vi "vi tree.vi"   [LabVIEW 2020, in "stream_custom_cluster.lvclass"]
uses:
  stream_custom_cluster.lvclass
  stream_custom_cluster.lvclass/stream_custom_cluster.ctl
  <userlib>/_OpenG.lib/lvdata/lvdata.llb/ClassLoader__ogtk.lvclass
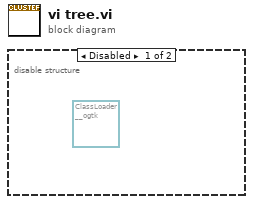
[diagram p0: block diagram]
diagram:
  n1 = disable-structure shown="Disabled" {
    frame Disabled {
      (unwired) refnum<class "ClassLoader__ogtk.lvclass"> refnum ("openg_variant.lvlib:ClassLoader__ogtk.lvclass")
    }
    frame Enabled {
    }
  }
